vi "串口工具.vi"() -> ()   [LabVIEW 2015]
uses:
  <vilib>/Platform/TimedLoop/XDataNode/timing_clust.ctl
  <vilib>/Platform/TimedLoop/XDataNode/nitl_modes.ctl
  <vilib>/Platform/TimedLoop/XDataNode/wakeup.ctl
  <vilib>/Instr/_visa.llb/VISA Configure Serial Port (Instr).vi
  <vilib>/Platform/TimedLoop/XDataNode/XDataNode.xnode
  <vilib>/Platform/TimedLoop/XDataNode/XDNodeRunTimeDep.lvlib
panel:
  in  "清空":bool
  in  "停止":bool
  in  "暂停/恢复":bool
  out "读取缓冲区":string
  out "返回数":u32
  in  "baud rate (115200)":u32=115200 caption="波特率(115200)"
  in  "VISA resource name":refnum<visa-resource-name> caption="串口"
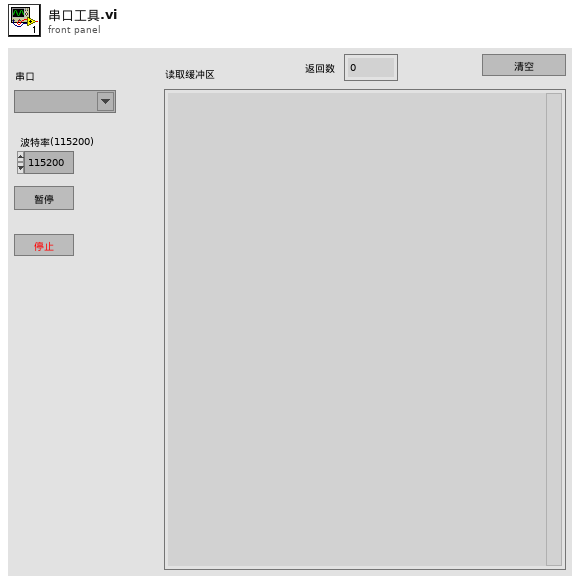
[diagram p1: front panel]
types:
  T1 = typedef "XDNodeRunTimeDep.lvlib/timing_clust.ctl" = cluster{"Expected End [f-1]":u64, "Actual End [f-1]":u64, "Finished Late? [f-1]":bool, "Expected End [i-1]":u64, "Actual End [i-1]":u64, "Finished Late? [i-1]":bool, "Expected Start [i]":u64, "Actual Start [i]":u64, "Expected Start [f]":u64, "Actual Start [f]":u64, "Source Name":string, "Structure Name":string, "Period":i64, "Deadline":i64, "Offset":i64, "Start":i64, "Priority":i32, "Timeout":i32, "Mode":T2, "Wakeup Reason":T3, "Error":errorcluster, "Source Type":string, "Secondary Source Type":string, "Global End Time":u64, "Global Start Time":u64, "Frame Duration":u64, "Iteration Duration":u64, "Assigned CPU":i32, "I/O Scan Engine Mode":u32}
  T2 = typedef "XDNodeRunTimeDep.lvlib/nitl_modes.ctl" = enum32{"No Change", "Process missed periods, maintain original phase", "Discard missed periods, maintain original phase", "Process missed periods, ignore original phase", "Discard missed periods, ignore original phase"}
  T3 = typedef "XDNodeRunTimeDep.lvlib/wakeup.ctl" = enum32{"Normal", "Aborted", "Asynchronous wakeup", "Timing source error", "Timed loop error", "Timeout"}
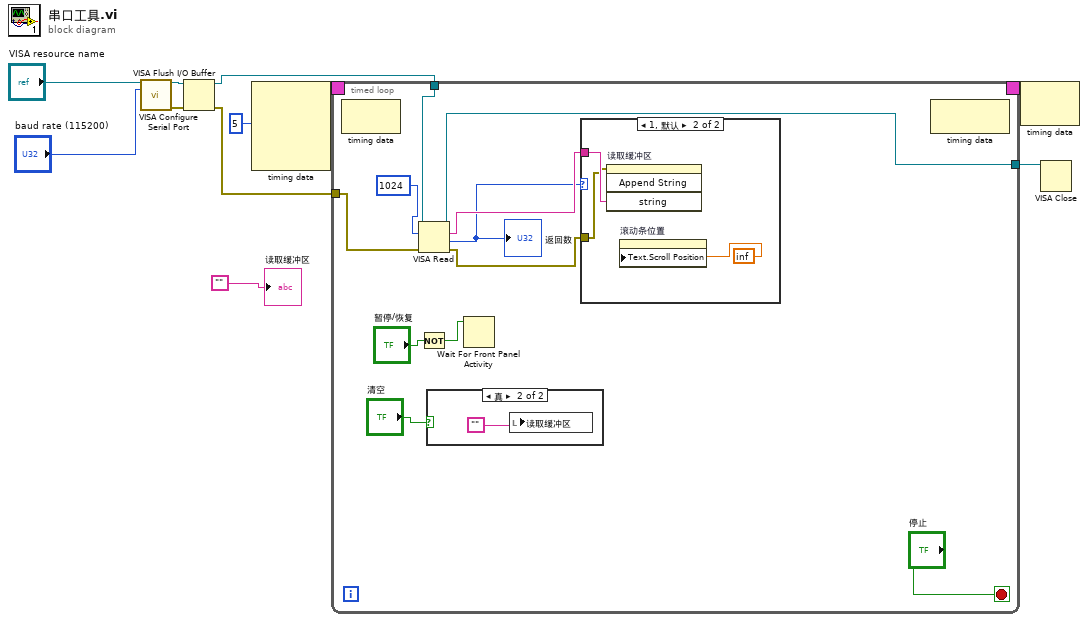
[diagram p0: block diagram]
diagram:
  n1 = call-poly "VISA Configure Serial Port"("VISA resource name"="VISA resource name", "baud rate (9600)"="baud rate (115200)") -> ("VISA resource name out"=w4:refnum<visa-resource-name>, "error out"=w3:errorcluster)  [unwired: 12 in]
  n2 = VISA Flush I/O Buffer(VISA resource name=w4, error in (no error)=w3) -> (VISA resource name out=w5:refnum<visa-resource-name>, error out=w2:errorcluster)  [unwired: 1 in]
  n3 = node-c288(i64 5 ("周期")) -> (w9:T1)  [unwired: 3 in]
  n4 = timed-loop {
    tunnel: w5 -> [w22]
    timing: w9 -> [_]
    timing-out: [_] -> w8
    tunnel: [w12] -> w6
    tunnel: w2 -> [w19]
    stop <- "停止" stop-if-true
    n5 = node-c288() -> ()  [unwired: 1 in, 1 out]
    n6 = VISA Read(VISA resource name=w22, byte count=u32 1024 ("字节总数"), error in (no error)=w19) -> (VISA resource name out=w12:refnum<visa-resource-name>, read buffer=w20:string, return count=w17:u32, error out=w21:errorcluster)
    "返回数" <- w17
    n7 = Not(x="暂停/恢复") -> (.not. x?=w14:bool)
    n8 = case shown="真" "清空" {
      frame False {
      }
      frame True {
        n9 = local write "读取缓冲区"("") -> ()
      }
    }
    n10 = Wait For Front Panel Activity(3:w14) -> ()  [unwired: 2 in, 1 out]
    n11 = case shown="1, 默认" w17 {
      tunnel: w20 -> [_ w28]
      tunnel: w21 -> [_ w27]
      frame 0 {
      }
      frame 1, Default {
        n12 = invoke on="读取缓冲区" class="Str" method="Append String"(error in=w27, "string"=w28) -> ()  [unwired: 2 in, 4 out]
        n13 = property on="滚动条位置" class="Str"("Text.Scroll Position"=inf) -> ()  [unwired: 2 in, 2 out]
      }
    }
    n14 = node-c288() -> ()  [unwired: 1 in, 1 out]
  }
  n15 = node-c288(w8) -> ()  [unwired: 1 out]
  n16 = VISA Close(VISA resource name=w6) -> ()  [unwired: 1 in, 1 out]
  "读取缓冲区" <- ""
